vi "Read Structure.vi"(8 "error in (no error)":errorcluster, 11 "Structures in":refnum<class "Structures.lvclass">) -> (0 "error out":errorcluster, 2 "Structure":refnum<vi>, 3 "Structures out":refnum<class "Structures.lvclass">)   [LabVIEW 2019, in "Structures.lvclass"]
uses:
  Structures.lvclass
  Structures.lvclass/Structures.ctl
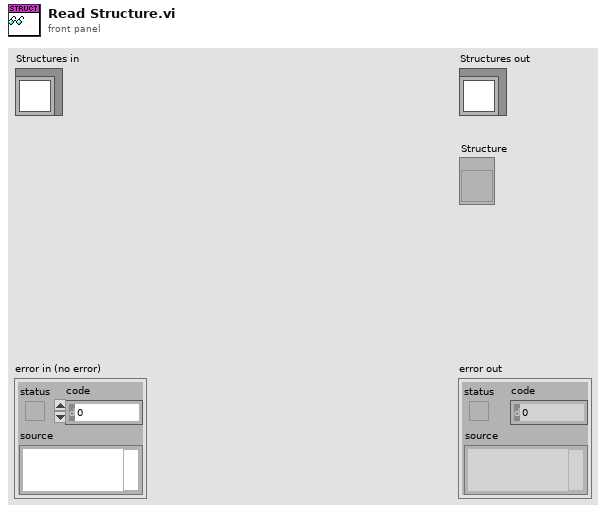
[diagram p1: front panel]
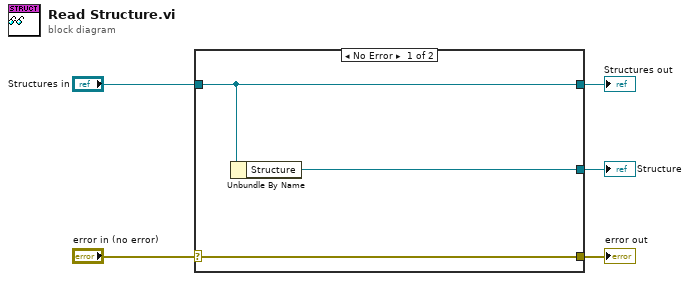
[diagram p0: block diagram]
diagram:
  n1 = case shown="No Error" "error in (no error)" {
    selector: "error in (no error)" -> [w8 w9]
    tunnel: [w8 w9] -> w4
    tunnel: [w7 w10] -> w2
    tunnel: "Structures in" -> [w7 w10]
    tunnel: [w6 _] -> w1
    frame No Error {
      n2 = Unbundle By Name(w7) -> ("Structure"=w6:refnum<vi>)
    }
    frame Error {
    }
  }
  "error out" <- w4
  "Structures out" <- w2
  "Structure" <- w1
